vi "Oclaro_FB_INJ.vi"(1 "Resistance (k Ohms)":dbl=10.0) -> ()   [LabVIEW 2014]
doc: "Use this template to measure or generate signals using the DAQ Assistant Express VI and NI-DAQmx. Double click the DAQ Assistant Express VI to launch a configuration wizard which steps you through configuring a measurement or generation.\n\nNote: You must have an NI-DAQmx compatible device installed to use this Express VI. Refer to the DAQ Quick Start Guide for NI-DAQ 7.0 for a list of compatible devices."
uses:
  <vilib>/addons/zeromq/socket_type.ctl
  Instance           8 18Saved   INJ FB Map .vi
  <instrlib>/Tektronix 7000 Series/Public/Data/Read (Single Waveform).vi
  <instrlib>/Tektronix 7000 Series/Tektronix 7000 Series.lvlib
  <vilib>/addons/zeromq/zeromq.lvlib
  <vilib>/addons/zeromq/zmq_context.lvclass
  <vilib>/addons/zeromq/zmq_socket.lvclass
panel:
  out "Status":string="Complete"
  out "Start time":timestamp=timestamp(3444094609.1761975 s since 1904-01-01)
  in  "Current Source Address":refnum<visa-resource-name>="GPIB0::3::INSTR"
  in  "TEC Address":refnum<visa-resource-name>="GPIB0::2::INSTR"
  in  "Channel (0: Channel 1)":u16(ring)=2 format="%#_5f" items=["Channel 1", "Channel 2", "Channel 3", "Channel 4", "Math 1", "Math 2", "Math 3", "Math 4", "Reference 1", "Reference 2", "Reference 3", "Reference 4"]
  out "Total Time (hrs)":dbl=9.063415388796065
  out "Finish time":timestamp=timestamp(3444066478.193819 s since 1904-01-01)
  in  "Tek Scope Address":refnum<visa-resource-name>="GPIB0::4::INSTR"
  in  "Time to wait for TEC (sec)":dbl=15.0 caption="Delay Time (s)"
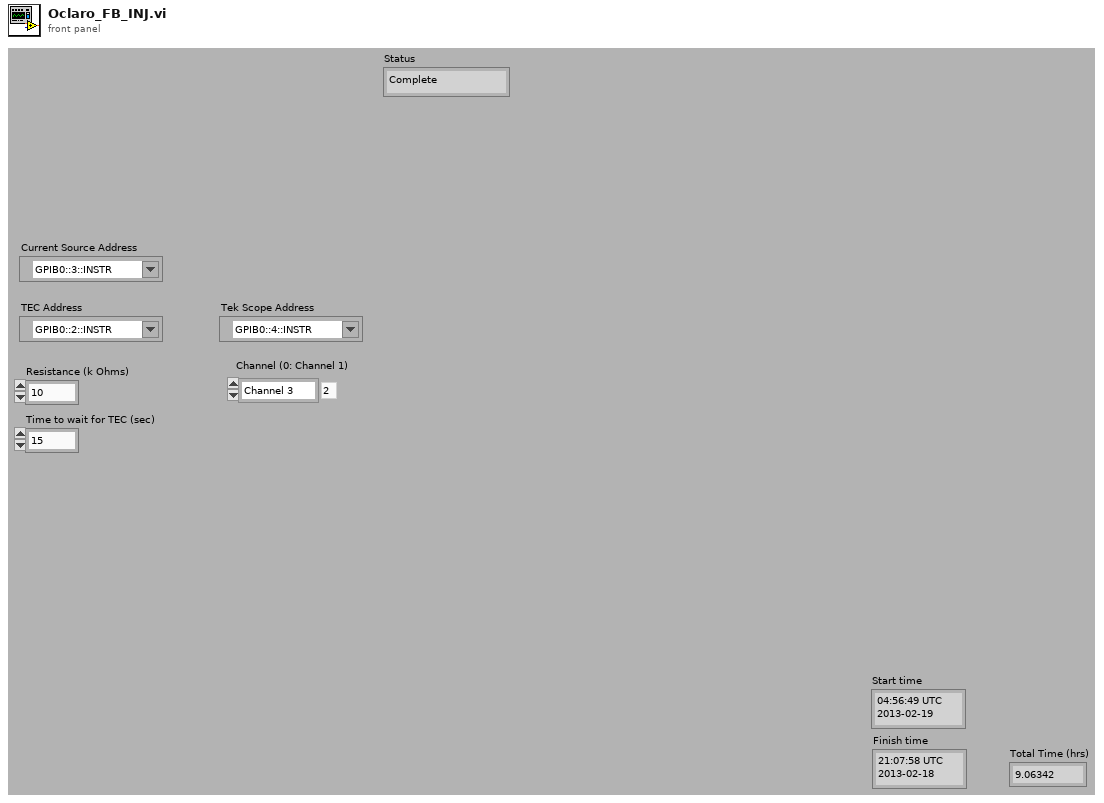
[diagram p1: front panel]
types:
  T1 = typedef "zeromq.lvlib/socket_type.ctl" = enum8{"ZMQ_PAIR", "ZMQ_PUB", "ZMQ_SUB", "ZMQ_REQ", "ZMQ_REP", "ZMQ_DEALER", "ZMQ_ROUTER", "ZMQ_PULL", "ZMQ_PUSH", "ZMQ_XPUB", "ZMQ_XSUB"}
  T2 = enum16{"big-endian, network order", "native, host order", "little-endian"}
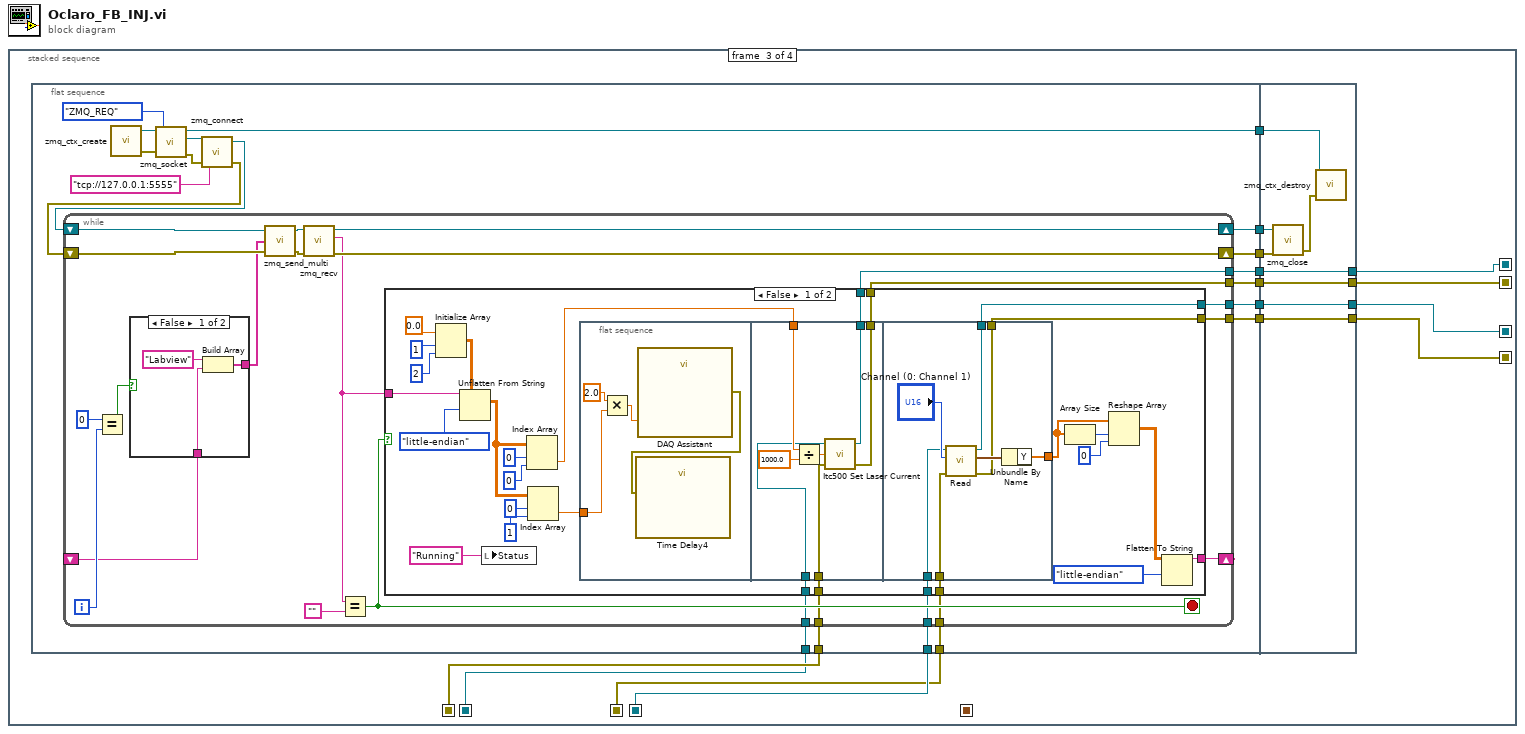
[diagram p0: block diagram]
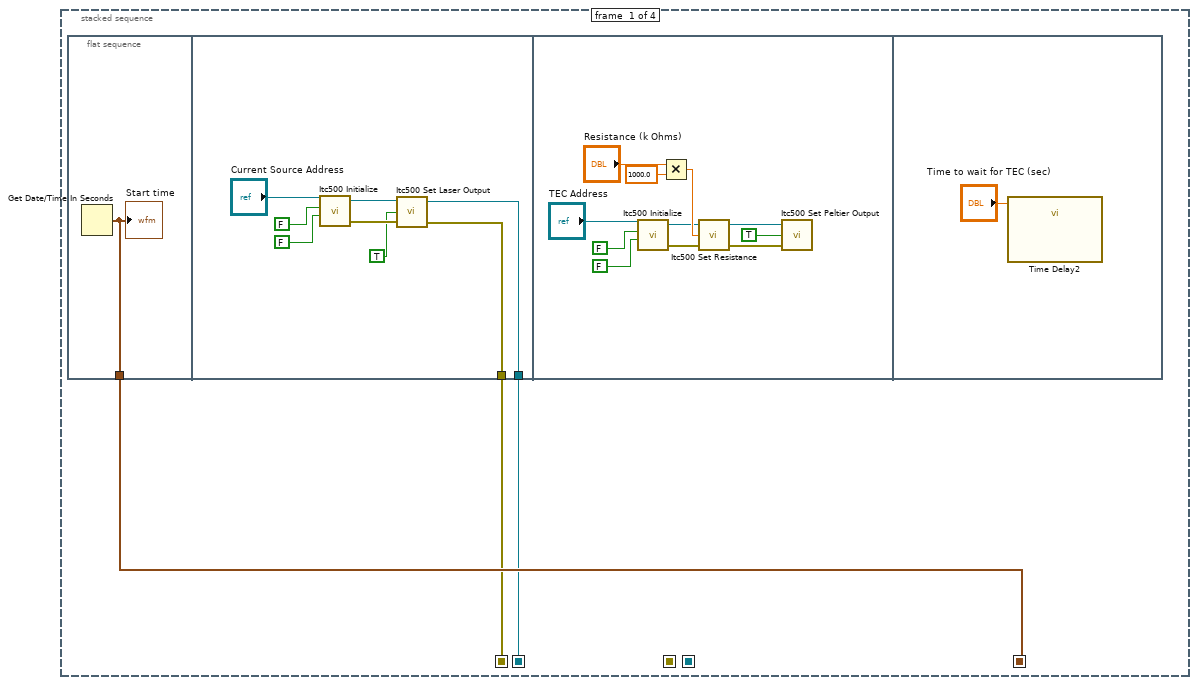
[diagram p2: hidden frame]
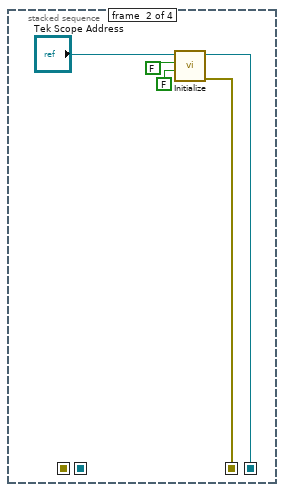
[diagram p3: hidden frame]
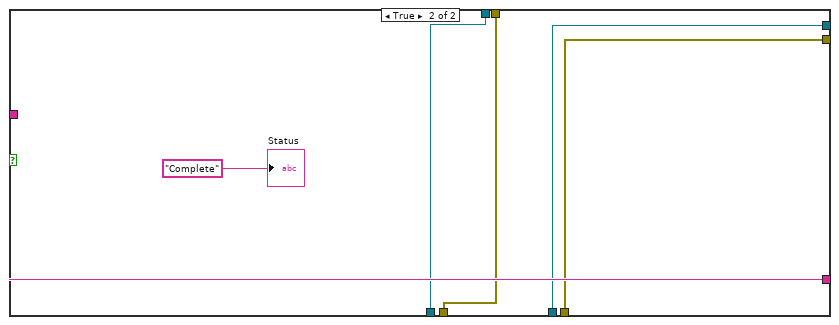
[diagram p4: hidden frame]
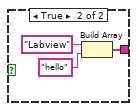
[diagram p5: hidden frame]
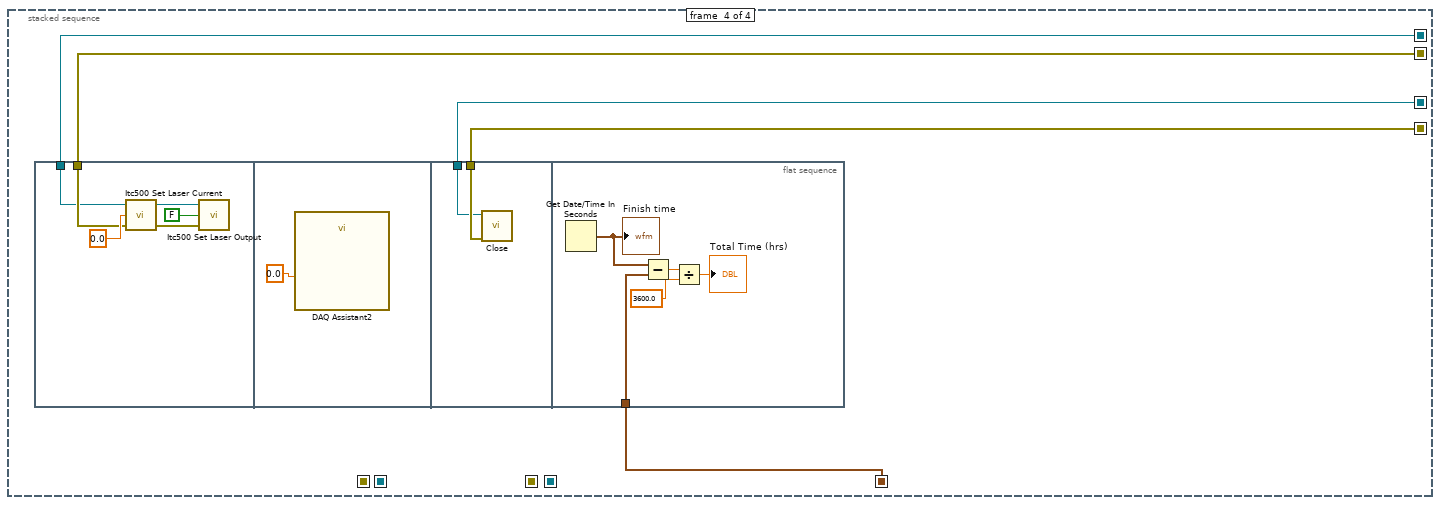
[diagram p6: hidden frame]
diagram:
  n1 = stacked-sequence {
    seq-local: [_ w25 _ _] -> [_ _ w38 _]
    seq-local: [_ w26 _ _] -> [_ _ w39 _]
    seq-local: [_ _ w30 _] -> [_ _ _ w156]
    seq-local: [_ _ w32 _] -> [_ _ _ w157]
    seq-local: [w3 _ _ _] -> [_ _ _ w153]
    seq-local: [_ _ w34 _] -> [_ _ _ w154]
    seq-local: [_ _ w36 _] -> [_ _ _ w155]
    seq-local: [w1 _ _ _] -> [_ _ w40 _]
    seq-local: [w2 _ _ _] -> [_ _ w41 _]
    frame #0 {
      n2 = flat-sequence {
        tunnel: [w4] -> w3
        tunnel: [w6] -> w2
        tunnel: [w5] -> w1
        frame #0 {
          n3 = Get Date/Time In Seconds() -> (seconds since 1Jan1904=w4:timestamp)
          "Start time" <- w4
        }
        frame #1 {
          n4 = call <instrlib>:"Itc500 Initialize.vi"("reset device"=FALSE, "id query"=FALSE, "resource name"="Current Source Address") -> ("error out"=w12:errorcluster, "instrument handle"=w11:refnum<visa-resource-name>)  [unwired: 1 in, 1 out]
          n5 = call <instrlib>:"Itc500 Set Laser Output.vi"("error in (no error)"=w12, "output"=TRUE, "instrument handle"=w11) -> ("error out"=w6:errorcluster, "instrument handle out"=w5:refnum<visa-resource-name>)  [unwired: 1 out]
        }
        frame #2 {
          n6 = call <instrlib>:"Itc500 Initialize.vi"("reset device"=FALSE, "id query"=FALSE, "resource name"="TEC Address") -> ("error out"=w19:errorcluster, "instrument handle"=w18:refnum<visa-resource-name>)  [unwired: 1 in, 1 out]
          n7 = Multiply(x="Resistance (k Ohms)", y=1000.0) -> (x*y=w22:dbl)
          n8 = call <instrlib>:"Itc500 Set Resistance.vi"("error in (no error)"=w19, "resistance"=w22, "instrument handle"=w18) -> ("error out"=w16:errorcluster, "instrument handle out"=w15:refnum<visa-resource-name>)  [unwired: 1 out]
          n9 = call <instrlib>:"Itc500 Set Peltier Output.vi"("error in (no error)"=w16, "output"=TRUE, "instrument handle"=w15) -> ()  [unwired: 3 out]
        }
        frame #3 {
          n10 = call "Time Delay2"("Delay Time (s)"="Time to wait for TEC (sec)") -> ()  [unwired: 10 in, 1 out]
        }
      }
    }
    frame #1 {
      n11 = call <instrlib>:"Initialize.vi"("Reset? ( Yes)"=FALSE ("Reset (T: Reset)"), "ID Query? ( Yes)"=FALSE ("Reset (T: Reset)"), "VISA resource name"="Tek Scope Address") -> ("error out"=w25:errorcluster, "VISA resource name out"=w26:refnum<visa-resource-name>)  [unwired: 7 in]
    }
    frame #2 {
      n12 = flat-sequence {
        tunnel: [w59] -> w44
        tunnel: [w53] -> w43
        tunnel: [w54] -> w42
        tunnel: w41 -> [w52]
        tunnel: w40 -> [w51]
        tunnel: w39 -> [w50]
        tunnel: w38 -> [w49]
        tunnel: [w48] -> w37
        tunnel: [w47] -> w35
        tunnel: [w46] -> w33
        tunnel: [w45] -> w31
        tunnel: w44 -> [w152]
        tunnel: w43 -> [w150]
        tunnel: w42 -> [w149]
        tunnel: [w148] -> w36
        tunnel: w37 -> [w148]
        tunnel: [w147] -> w34
        tunnel: w35 -> [w147]
        tunnel: [w146] -> w32
        tunnel: w33 -> [w146]
        tunnel: [w145] -> w30
        tunnel: w31 -> [w145]
        frame #0 {
          n13 = call <vilib>:"zmq_ctx_create.vi"() -> ("error out"=w58:errorcluster, "context out"=w63:refnum<class "zmq_context.lvclass">)  [unwired: 4 in]
          n14 = call <vilib>:"zmq_socket.vi"("error in"=w58, "socket type"=socket_type."ZMQ_REQ", "context in"=w63) -> ("error out"=w62:errorcluster, "socket out"=w61:refnum<class "zmq_socket.lvclass">, "context out"=w59:refnum<class "zmq_context.lvclass">)  [unwired: 2 in]
          n15 = call <vilib>:"zmq_connect.vi"("error in"=w62, "endpoint"="tcp://127.0.0.1:5555", "socket in"=w61) -> ("error out"=w55:errorcluster, "socket out"=w60:refnum<class "zmq_socket.lvclass">)  [unwired: 1 in]
          n16 = while {
            shift-right: [w81] -> w53
            shift-left: w60 -> [w86]
            shift-right: [w82] -> w54
            shift-left: w55 -> [w85]
            shift-right: [w80] -> _
            shift-left: _ -> [w76]
            tunnel: w52 -> [w71]
            tunnel: w51 -> [w70]
            tunnel: w50 -> [w69]
            tunnel: w49 -> [w68]
            tunnel: [w67] -> w48
            tunnel: [w66] -> w47
            tunnel: [w65] -> w46
            tunnel: [w64] -> w45
            i -> [w79]
            stop <- w73 stop-if-true
            n17 = Equal?(x=0, y=w79) -> (x = y?=w77:bool)
            n18 = case shown="False" w77 {
              tunnel: [w140 w144] -> w72
              tunnel: w76 -> [w139 _]
              frame False {
                n19 = Build Array("Labview", w139) -> (w140:string[])
              }
              frame True {
                n20 = Build Array("Labview", "hello" ("element")) -> (w144:string[])
              }
            }
            n21 = call <vilib>:"zmq_send_multi.vi"("error in"=w85, "parts"=w72, "socket in"=w86) -> ("error out"=w83:errorcluster, "socket out"=w84:refnum<class "zmq_socket.lvclass">)  [unwired: 1 in]
            n22 = call <vilib>:"zmq_recv.vi"("error in"=w83, "socket in"=w84) -> ("error out"=w82:errorcluster, "data"=w74:string, "socket out"=w81:refnum<class "zmq_socket.lvclass">)  [unwired: 3 in, 2 out]
            n23 = Equal?(x=w74, y="") -> (x = y?=w73:bool)
            n24 = case shown="False" w73 {
              tunnel: [w103 w138] -> w80
              tunnel: w74 -> [w102 w138]
              tunnel: w71 -> [w94 w135]
              tunnel: w70 -> [w93 w136]
              tunnel: w69 -> [w92 w134]
              tunnel: w68 -> [w91 w133]
              tunnel: [w90 w133] -> w67
              tunnel: [w89 w134] -> w66
              tunnel: [w88 w136] -> w64
              tunnel: [w87 w135] -> w65
              frame False {
                n25 = Initialize Array(0.0, 1 ("dimension size"), 2 ("dimension size")) -> (w110:dbl[][])
                n26 = Unflatten From String(type=w110, binary string=w102, byte order (0:big-endian, network order)=T2."little-endian") -> (value=w107:dbl[][])  [unwired: 2 in, 2 out]
                n27 = local write "Status"("Running" ("Status")) -> ()
                n28 = Index Array(array=w107, index (row)=0 ("disabled index (row)"), index (col)=0 ("disabled index (col)")) -> (element=w99:dbl)
                n29 = Index Array(array=w107, index (row)=0 ("disabled index (row)"), index (col)=1 ("disabled index (col)")) -> (element=w100:dbl)
                n30 = flat-sequence {
                  tunnel: w100 -> [w115]
                  tunnel: w99 -> [w123]
                  tunnel: w94 -> [w122]
                  tunnel: w93 -> [w121]
                  tunnel: [w120] -> w88
                  tunnel: [w119] -> w87
                  tunnel: [w130] -> w97
                  tunnel: w92 -> [w129]
                  tunnel: w91 -> [w128]
                  tunnel: [w127] -> w89
                  tunnel: [w126] -> w90
                  frame #0 {
                    n31 = Multiply(x=2.0, y=w115) -> (x*y=w118:dbl)
                    n32 = call "DAQ Assistant"("data"=w118) -> ("error out"=w116:errorcluster)  [unwired: 17 in, 1 out]
                    n33 = call "Time Delay4"("error in (no error)"=w116) -> ()  [unwired: 10 in, 1 out]
                  }
                  frame #1 {
                    n34 = Divide(x=w123, y=1000.0) -> (x/y=w124:dbl)
                    n35 = call <instrlib>:"Itc500 Set Laser Current.vi"("error in (no error)"=w122, "current"=w124, "instrument handle"=w121) -> ("error out"=w119:errorcluster, "instrument handle out"=w120:refnum<visa-resource-name>)  [unwired: 1 out]
                  }
                  frame #2 {
                    n36 = call-poly <instrlib>:"Read.vi"("error in (no error)"=w128, "Channel (0: Channel 1)"="Channel (0: Channel 1)", "VISA resource name"=w129) -> ("error out"=w126:errorcluster, "Waveform Data"=w132:waveform(dbl), "VISA resource name out"=w127:refnum<visa-resource-name>)  [unwired: 6 in]
                    n37 = Unbundle By Name(w132) -> ("Y"=w130:dbl[])
                  }
                }
                n38 = Array Size(array=w97) -> (size(s)=w96:i32)
                n39 = Reshape Array(w97, w96, 0 ("dimension size")) -> (w95:dbl[][])
                n40 = Flatten To String(anything=w95, byte order (0:big-endian, network order)=T2."little-endian") -> (data string=w103:string)  [unwired: 2 in, 2 out]
              }
              frame True {
                "Status" <- "Complete"
              }
            }
          }
        }
        frame #1 {
          n41 = call <vilib>:"zmq_close.vi"("error in"=w149, "socket"=w150) -> ("error out"=w151:errorcluster)  [unwired: 3 in]
          n42 = call <vilib>:"zmq_ctx_destroy.vi"("error in"=w151, "context in"=w152) -> ()  [unwired: 3 in, 1 out]
        }
      }
    }
    frame #3 {
      n43 = flat-sequence {
        tunnel: w157 -> [w159]
        tunnel: w156 -> [w158]
        tunnel: w155 -> [w166]
        tunnel: w154 -> [w165]
        tunnel: w153 -> [w167]
        frame #0 {
          n44 = call <instrlib>:"Itc500 Set Laser Current.vi"("error in (no error)"=w159, "current"=0.0, "instrument handle"=w158) -> ("error out"=w162:errorcluster, "instrument handle out"=w161:refnum<visa-resource-name>)  [unwired: 1 out]
          n45 = call <instrlib>:"Itc500 Set Laser Output.vi"("error in (no error)"=w162, "output"=FALSE, "instrument handle"=w161) -> ()  [unwired: 3 out]
        }
        frame #1 {
          n46 = call "DAQ Assistant2"("data"=0.0) -> ()  [unwired: 17 in, 2 out]
        }
        frame #2 {
          n47 = call <instrlib>:"Close.vi"("error in (no error)"=w166, "VISA resource name"=w165) -> ()  [unwired: 9 in, 1 out]
        }
        frame #3 {
          n48 = Get Date/Time In Seconds() -> (seconds since 1Jan1904=w168:timestamp)
          "Finish time" <- w168
          n49 = Subtract(x=w168, y=w167) -> (x-y=w170:dbl)
          n50 = Divide(x=w170, y=3600.0) -> (x/y=→"Total Time (hrs)":dbl)
        }
      }
    }
  }
